vi "Fetch Voltage.vi"(7 "Maximum Time (30000 ms)":u32=30000, 8 "error in (no error)":errorcluster, 9 "Measurement Number (\t1: Measurement 1)":u32(ring)=1 items=["Measurement 1"=1, "Measurement 2"=2, "Measurement 3"=3, "Measurement 4"=4], 10 "Voltage Name (0: V0)":u32(ring) items=["V0", "V1", "VCMP0", "VCMP1", "VRF0", "VRF1", "PV1"], 11 "VISA resource name":refnum<visa-resource-name>) -> (0 "error out":errorcluster, 2 "Measurement Data":dbl, 3 "VISA resource name out":refnum<visa-resource-name>)   [LabVIEW 2011, in "Agilent N432A.lvlib"]
doc: "Fetches the measurement data of V0, V1 VCMP0, VCMP1, VRF0, VRF1 or PV1 for the specified window/measurement. You need to initiate an acquisition with the Initiate VI prior to calling this VI.\n\n<B>Note:</B>\n\nYou must use the Configure Measurement.vi and Configure Relative Measurement.vi to set the power meter before using this VI to fetch data.\n\nUse this VI only with other low-level VIs. The high-level VIs automatically incorporate this functionality. This VI does not check the instrument status."
uses:
  <instrlib>/Agilent N432A/Agilent N432A.lvlib
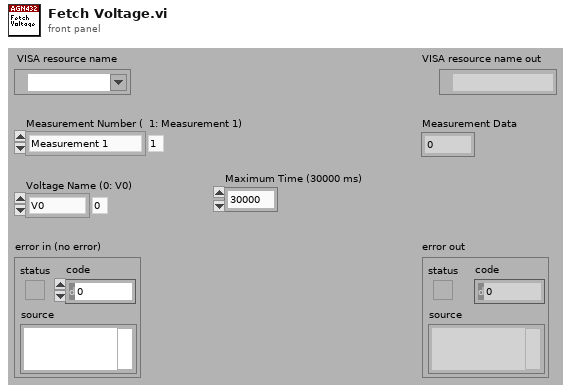
[diagram p1: front panel]
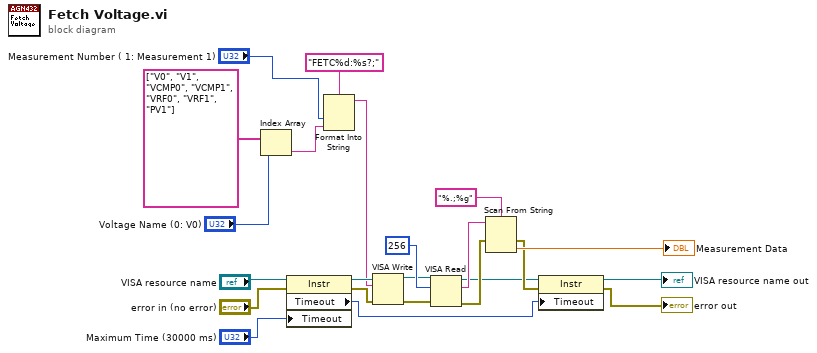
[diagram p0: block diagram]
diagram:
  n1 = Index Array(array=string[] ["V0", "V1", "VCMP0", "VCMP1", "VRF0", "VRF1", "PV1"], index="Voltage Name (0: V0)") -> (element=w19:string)
  n2 = property class="Instr"(reference="VISA resource name", error in="error in (no error)", "Timeout"="Maximum Time (30000 ms)") -> (reference out=w14:refnum<visa-resource-name>, error out=w15:errorcluster, "Timeout"=w3:u32)
  n3 = Format Into String(format string="FETC%d:%s?;", "Measurement Number (\t1: Measurement 1)", w19) -> (resulting string=w13:string)  [unwired: 2 in, 1 out]
  n4 = VISA Write(VISA resource name=w14, write buffer=w13, error in (no error)=w15) -> (VISA resource name out=w11:refnum<visa-resource-name>, error out=w10:errorcluster)  [unwired: 1 out]
  n5 = VISA Read(VISA resource name=w11, byte count=u32 256, error in (no error)=w10) -> (VISA resource name out=w4:refnum<visa-resource-name>, read buffer=w8:string, error out=w5:errorcluster)  [unwired: 1 out]
  n6 = Scan From String(format string="%.;%g", input string=w8, error in=w5) -> (error out=w6:errorcluster, output 1=→"Measurement Data":dbl)  [unwired: 2 in, 2 out]
  n7 = property class="Instr"(reference=w4, error in=w6, "Timeout"=w3) -> (reference out=→"VISA resource name out":refnum<visa-resource-name>, error out=→"error out":errorcluster)
